vi "getFilename.vi"(11 "Extension":string) -> (3 "Filename":path)   [LabVIEW 2012]
uses:
  variables/GlobalUI.vi
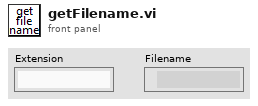
[diagram p1: front panel]
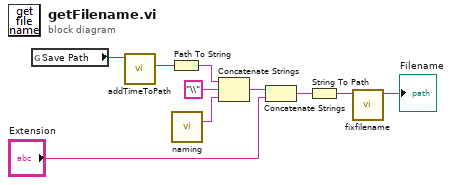
[diagram p0: block diagram]
diagram:
  n1 = global read "GlobalUI.vi" "Save Path"() -> (w2:path)
  n2 = call "addTimeToPath.vi"("Path"=w2) -> ("Time Path (Path)"=w1:path)  [unwired: 9 in, 1 out]
  n3 = Path To String(path=w1) -> (string=w6:string)
  n4 = call "naming.vi"() -> ("filename"=w3:string)  [unwired: 15 in]
  n5 = Concatenate Strings(w6, "\\" ("string"), w3) -> (w4:string)
  n6 = Concatenate Strings(w4, "Extension") -> (w9:string)
  n7 = String To Path(string=w9) -> (path=w8:path)
  n8 = call "fixfilename.vi"("Path"=w8) -> ("fixed path"=→"Filename":path)  [unwired: 9 in, 1 out]
